vi "SSP - get header (listbox).vi"(8 "error in (no error)":errorcluster, 11 "JSON string":string) -> (0 "error out":errorcluster, 3 "value":string)   [LabVIEW 2020, in "ui-testing.lvlib"]
doc: "copyright: Thomas Zilliox©"
uses:
  ui-testing.lvlib
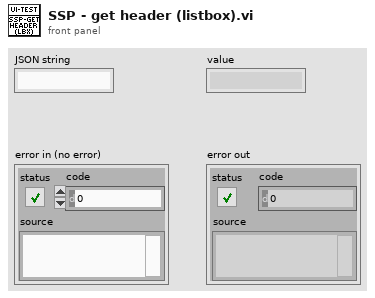
[diagram p1: front panel]
types:
  T1 = cluster{"control":string, "subpanel":string, "subsubpanel":string}
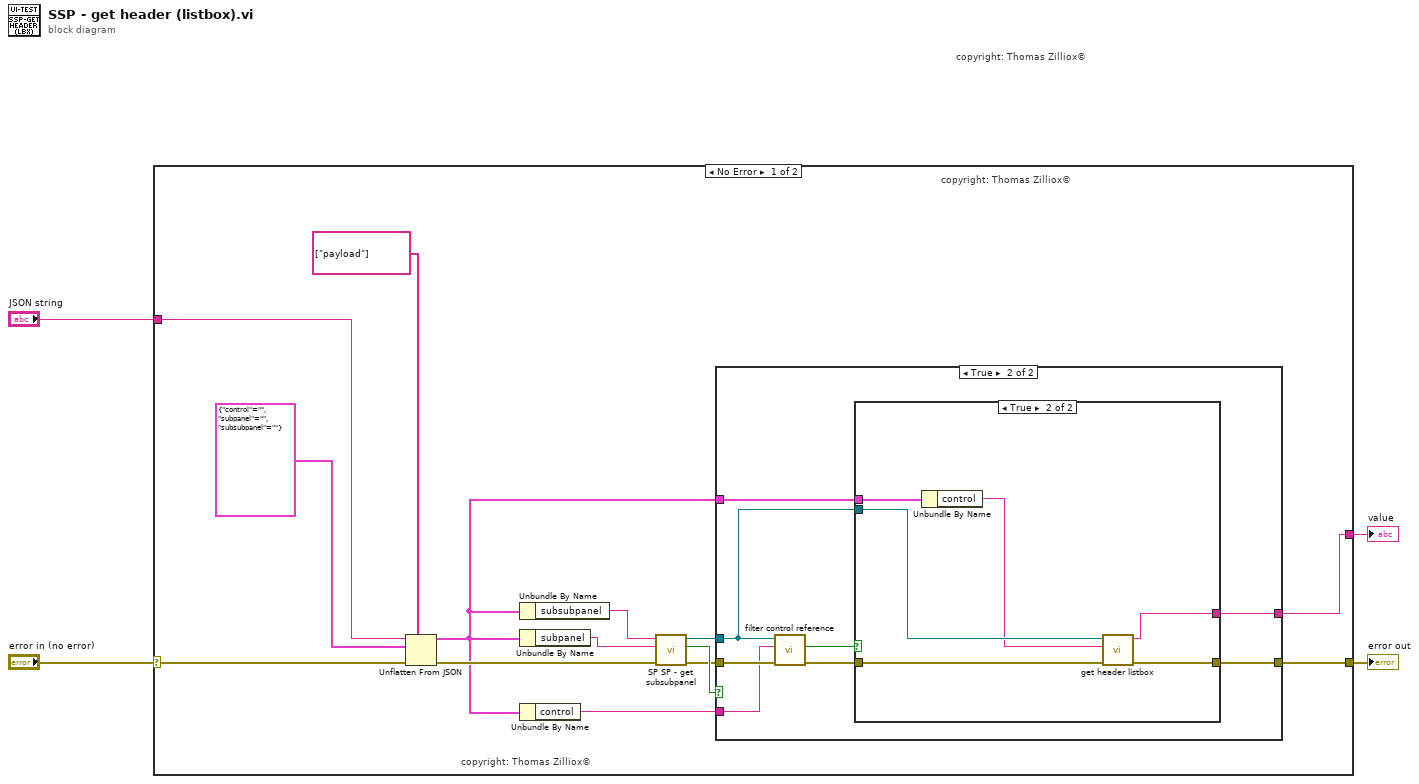
[diagram p0: block diagram]
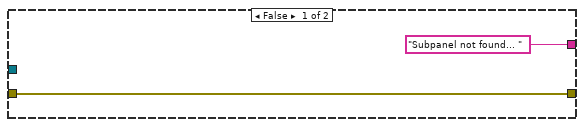
[diagram p2: hidden frame]
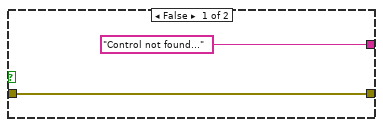
[diagram p3: hidden frame]
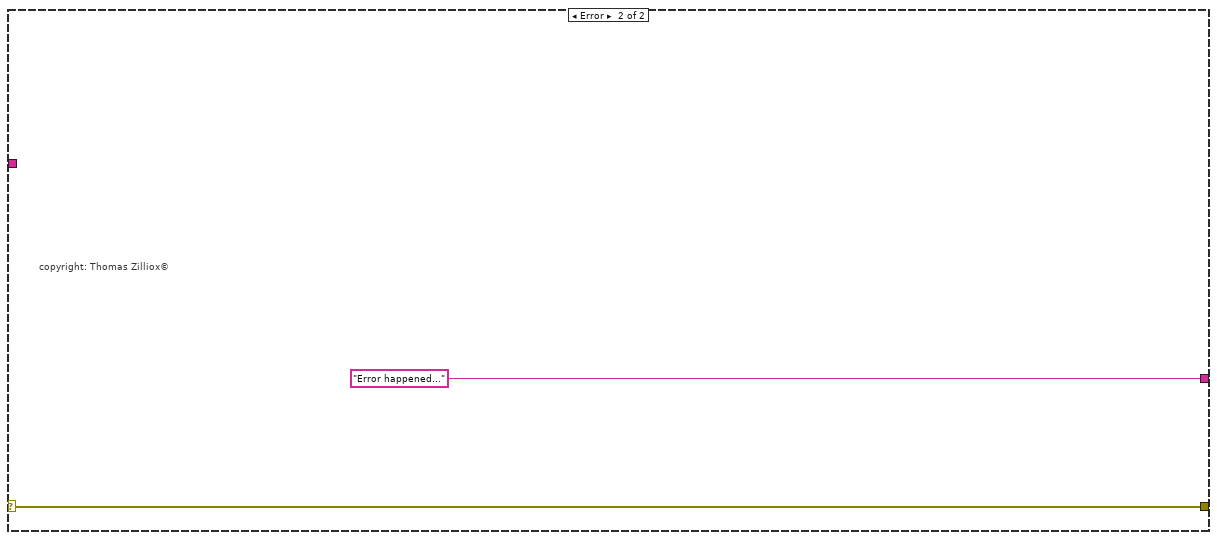
[diagram p4: hidden frame]
diagram:
  # "copyright: Thomas Zilliox©"
  n1 = case shown="No Error" "error in (no error)" {
    selector: "error in (no error)" -> [w8 w38]
    tunnel: "JSON string" -> [w5 _]
    tunnel: [w7 w38] -> w3
    tunnel: [w6 "Error happened..."] -> w2
    frame No Error {
      # "copyright: Thomas Zilliox©"
      # "copyright: Thomas Zilliox©"
      n2 = Unflatten From JSON(path=string[] ["payload"], JSON string=w5, type and defaults=T1 {"control"="", "subpanel"="", "subsubpanel"=""}, error in (no error)=w8) -> (value=w10:T1, error out=w17:errorcluster)  [unwired: 3 in]
      n3 = Unbundle By Name(w10) -> ("subsubpanel"=w9:string)
      n4 = Unbundle By Name(w10) -> ("subpanel"=w16:string)
      n5 = Unbundle By Name(w10) -> ("control"=w13:string)
      n6 = call "SP SP - get subsubpanel.vi"("error in (no error)"=w17, "subpanel"=w16, "subsubpanel"=w9) -> ("error out"=w11:errorcluster, "SubSubPanel found"=w12:bool, "SubSubPanel VI"=w14:refnum<vi>)  [unwired: 5 in, 1 out]
      n7 = case shown="True" w12 {
        tunnel: [w20 w28] -> w7
        tunnel: w14 -> [_ w25]
        tunnel: w11 -> [w20 w24]
        tunnel: w13 -> [_ w23]
        tunnel: ["Subpanel not found... " ("result string") w27] -> w6
        tunnel: w10 -> [_ w26]
        frame False {
        }
        frame True {
          n8 = call "filter control reference.vi"("error in (no error)"=w24, "Control label"=w23, "VI (Caller)"=w25) -> ("error out"=w21:errorcluster, "Control found"=w22:bool)  [unwired: 6 in, 1 out]
          n9 = case shown="True" w22 {
            tunnel: w21 -> [w30 w33]
            tunnel: [w30 w32] -> w28
            tunnel: ["Control not found..." ("result string") w31] -> w27
            tunnel: w26 -> [_ w36]
            tunnel: w25 -> [_ w35]
            frame False {
            }
            frame True {
              n10 = Unbundle By Name(w36) -> ("control"=w34:string)
              n11 = call "get header listbox.vi"("error in (no error)"=w33, "Control label"=w34, "VI (Caller)"=w35) -> ("error out"=w32:errorcluster, "headers"=w31:string)  [unwired: 7 in]
            }
          }
        }
      }
    }
    frame Error {
      # "copyright: Thomas Zilliox©"
    }
  }
  "error out" <- w3
  "value" <- w2
